vi "SerialPort.Function_Config Port Name.vi"(5 "Timeout(ms)":i32=1000, 7 "Module Name":string="Serial Port", 8 "error in":errorcluster, 10 "Com Port":string="COM4", 11 "Q In":refnum<queue>) -> (0 "error out":errorcluster)   [LabVIEW 2018]
uses:
  <vilib>/KATE/Queues/Q.Element.ctl
  <vilib>/KATE/Queues/Queue Utils.lvlib
panel:
  # "Serial Port - Set Com Port Name"
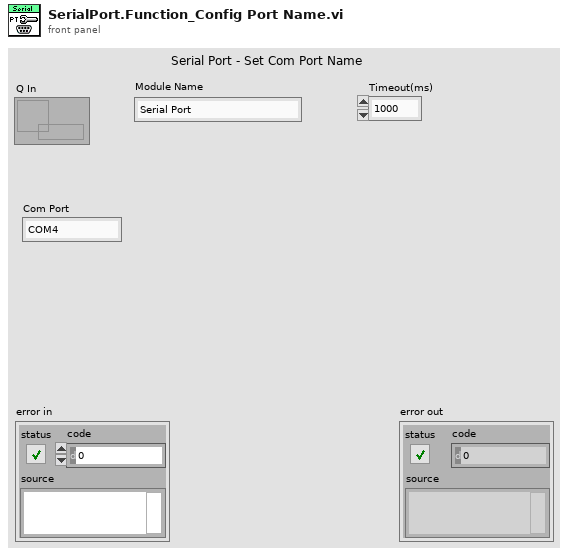
[diagram p1: front panel]
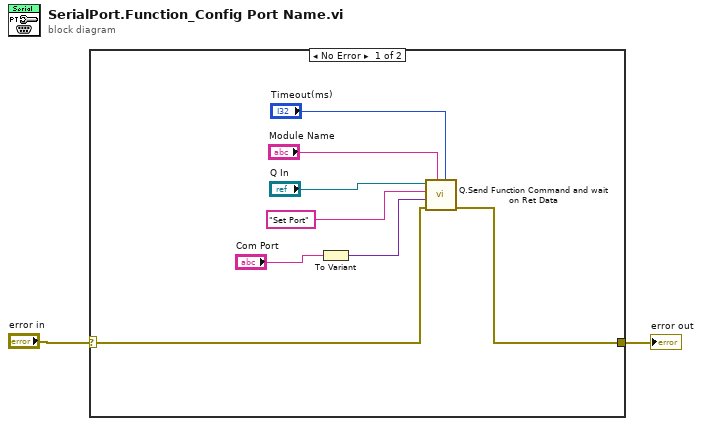
[diagram p0: block diagram]
diagram:
  n1 = case shown="No Error" "error in" {
    selector: "error in" -> [w6 w11]
    tunnel: [w5 w11] -> w1
    frame No Error {
      n2 = To Variant(anything="Com Port") -> (Variant=w4:variant)
      n3 = call <vilib>:"Q.Send Function Command and wait on Ret Data.vi"("Timeout(ms)"="Timeout(ms)", "Q Name"="Module Name", "error in"=w6, "Data1"=w4, "Cmd"="Set Port", "Q In"="Q In") -> ("error out"=w5:errorcluster)  [unwired: 4 in, 1 out]
    }
    frame Error {
    }
  }
  "error out" <- w1
